vi "SUB-FILE-Measurement data_Load.vi"(7 "File Name":string="Temperature", 8 "File Server Path":string="C:\\InLCT\\Measurement Data\\WB1\\1111\\PT") -> (1 "배열-Data":dbl[][](array[numeric])=[[30.4, 28.4, 28.4, 28.4, 28.4, 28.4, 28.4, 28.4, 28.4, 28.4, 28.4, 28.4, 28.4, 28.4, 28.4, 28.4, 28.4, 28.4, 28.4, 28.4, 28.4, 28.4, 28.4, 28.4, 28.4, 28.4, 28.4, 28.4, 28.4, 28.4, 28.4, 28.4, 28.4, 28.4, 28.4, 28.4, 28.4, 28.4, 28.4, 28.4, 28.4, 28.4, 28.4, 28.4, 28.4, 28.4, 28.4, 28.4, 28.4, 28.4, 28.4, 28.4, 28.4, 28.4, 28.4, 28.4, 28.4, 28.4, 28.4, 28.4, 28.4, 28.4, 28.4, 28.4, 28.4, 28.4, 28.4, 28.4, 28.4, 28.4, 28.4, 28.4, 28.4, 28.4, 28.4, 28.4, 28.4, 28.4, 28.4, 28.4, 28.4, 28.4, 28.4, 28.4, 28.4, 28.4, 28.4, 28.4, 28.4, 28.4, 28.4, 28.4, 28.4, 28.4, 28.4, 28.4, 28.4, 28.4, 28.4, 28.4, 28.4, 28.4, 28.4, 28.4, 28.4, 28.4, 28.4, 28.4, 28.4, 28.4, 28.4, 28.4, 28.4, 28.4, 28.4, 28.4, 28.4, 28.4, 28.4, 28.4, 28.4, 28.4, 28.4, 28.4, 28.4, 28.4, 28.4, 28.4, 28.4, 28.4, 28.4, 28.4, 28.4, 28.4, 28.4, 28.4, 28.4, 28.4, 28.4, 28.4, 28.4, 28.4, 28.4, 28.4, 28.4, 28.4, 28.4, 28.4, 28.4, 28.4, 28.4, 28.4, 28.4, 28.4, 28.4, 28.4, 28.4, 28.4, 28.4, 28.4, 28.4, 28.4, 28.4, 28.4, 28.4, 28.4, 28.4, 28.4, 28.4, 28.4, 28.4, 28.4, 28.4, 28.4, 28.4, 28.4, 28.4, 28.4, 28.4, 28.4, 28.4, 28.4, 28.4, 28.4, 28.4, 28.4, 28.4, 28.4, 28.4, 28.4, 28.4, 28.4, 28.4, 28.4, 28.4, 28.4, 28.4, 28.4, 28.4, 28.4, 28.4, 28.4, 28.4, 28.4, 28.4, 28.4, 28.4, 28.4, 28.4, 28.4, 28.4, 28.4, 28.4, 28.4, 28.4, 28.4, 28.4, 28.4, 28.4, 28.4, 28.4, 28.4, 28.4, 28.4, 28.4, 28.4, 28.4, 28.4, 28.4, 28.4, 28.4, 28.4, 28.4, 28.4, 28.4, 28.4, 28.4, 28.4, 28.4, 28.4, 28.4, 28.4, 28.4, 28.4, 28.4, 28.4, 28.4, 28.4, 28.4, 28.4, 28.4, 28.4, 28.4, 28.4, 28.4, 28.4, 28.4, 28.4, 28.4, 28.4, 28.4, 28.4, 28.4, 28.4, 28.4, 28.4, 28.4, 28.4, 28.4, 28.4, 28.4, 28.4, 28.4, 28.4, 28.4, 28.4, 28.4, 28.4, 28.4, 28.4, 28.4, 28.4, 28.4, 28.4, 28.4, 28.4, 28.4, 28.4], [28.4, 28.4, 28.4, 28.4, 28.4, 28.4, 28.4, 28.4, 28.4, 28.4, 28.4, 28.4, 28.4, 28.4, 28.4, 28.4, 28.4, 28.4, 28.4, 28.4, 28.4, 28.4, 28.4, 28.4, 28.4, 28.4, 28.4, 28.4, 28.4, 28.4, 28.4, 28.4, 28.4, 28.4, 28.4, 28.4, 28.4, 28.4, 28.4, 28.4, 28.4, 28.4, 28.4, 28.4, 28.4, 28.4, 28.4, 28.4, 28.4, 28.4, 28.4, 28.4, 28.4, 28.4, 28.4, 28.4, 28.4, 28.4, 28.4, 28.4, 28.4, 28.4, 28.4, 28.4, 28.4, 28.4, 28.4, 28.4, 28.4, 28.4, 28.4, 28.4, 28.4, 28.4, 28.4, 28.4, 28.4, 28.4, 28.4, 28.4, 28.4, 28.4, 28.4, 28.4, 28.4, 28.4, 28.4, 28.4, 28.4, 28.4, 28.4, 28.4, 28.4, 28.4, 28.4, 28.4, 28.4, 28.4, 28.4, 28.4, 28.4, 28.4, 28.4, 28.4, 28.4, 28.4, 28.4, 28.4, 28.4, 28.4, 28.4, 28.4, 28.4, 28.4, 28.4, 28.4, 28.4, 28.4, 28.4, 28.4, 28.4, 28.4, 28.4, 28.4, 28.4, 28.4, 28.4, 28.4, 28.4, 28.4, 28.4, 28.4, 28.4, 28.4, 28.4, 28.4, 28.4, 28.4, 28.4, 28.4, 28.4, 28.4, 28.4, 28.4, 28.4, 28.4, 28.4, 28.4, 28.4, 28.4, 28.4, 28.4, 28.4, 28.4, 28.4, 28.4, 28.4, 28.4, 28.4, 28.4, 28.4, 28.4, 28.4, 28.4, 28.4, 28.4, 28.4, 28.4, 28.4, 28.4, 28.4, 28.4, 28.4, 28.4, 28.4, 28.4, 28.4, 28.4, 28.4, 28.4, 28.4, 28.4, 28.4, 28.4, 28.4, 28.4, 28.4, 28.4, 28.4, 28.4, 28.4, 28.4, 28.4, 28.4, 28.4, 28.4, 28.4, 28.4, 28.4, 28.4, 28.4, 28.4, 28.4, 28.4, 28.4, 28.4, 28.4, 28.4, 28.4, 28.4, 28.4, 28.4, 28.4, 28.4, 28.4, 28.4, 28.4, 28.4, 28.4, 28.4, 28.4, 28.4, 28.4, 28.4, 28.4, 28.4, 28.4, 28.4, 28.4, 28.4, 28.4, 28.4, 28.4, 28.4, 28.4, 28.4, 28.4, 28.4, 28.4, 28.4, 28.4, 28.4, 28.4, 28.4, 28.4, 28.4, 28.4, 28.4, 28.4, 28.4, 28.4, 28.4, 28.4, 28.4, 28.4, 28.4, 28.4, 28.4, 28.4, 28.4, 28.4, 28.4, 28.4, 28.4, 28.4, 28.4, 28.4, 28.4, 28.4, 28.4, 28.4, 28.4, 28.4, 28.4, 28.4, 28.4, 28.4, 28.4, 28.4, 28.4, 28.4, 28.4, 28.4, 28.4, 28.4, 28.4, 28.4, 28.4], [28.4, 28.4, 28.4, 28.4, 28.4, 28.4, 28.4, 28.4, 28.4, 28.4, 28.4, 28.4, 28.4, 28.4, 28.4, 28.4, 28.4, 28.4, 28.4, 28.4, 28.4, 28.4, 28.4, 28.4, 28.4, 28.4, 28.4, 28.4, 28.4, 28.4, 28.4, 28.4, 28.4, 28.4, 28.4, 28.4, 28.4, 28.4, 28.4, 28.4, 28.4, 28.4, 28.4, 28.4, 28.4, 28.4, 28.4, 28.4, 28.4, 28.4, 28.4, 28.4, 28.4, 28.4, 28.4, 28.4, 28.4, 28.4, 28.4, 28.4, 28.4, 28.4, 28.4, 28.4, 28.4, 28.4, 28.4, 28.4, 28.4, 28.4, 28.4, 28.4, 28.4, 28.4, 28.4, 28.4, 28.4, 28.4, 28.4, 28.4, 28.4, 28.4, 28.4, 28.4, 28.4, 28.4, 28.4, 28.4, 28.4, 28.4, 28.4, 28.4, 28.4, 28.4, 28.4, 28.4, 28.4, 28.4, 28.4, 28.4, 28.4, 28.4, 28.4, 28.4, 28.4, 28.4, 28.4, 28.4, 28.4, 28.4, 28.4, 28.4, 28.4, 28.4, 28.4, 28.4, 28.4, 28.4, 28.4, 28.4, 28.4, 28.4, 28.4, 28.4, 28.4, 28.4, 28.4, 28.4, 28.4, 28.4, 28.4, 28.4, 28.4, 28.4, 28.4, 28.4, 28.4, 28.4, 28.4, 28.4, 28.4, 28.4, 28.4, 28.4, 28.4, 28.4, 28.4, 28.4, 28.4, 28.4, 28.4, 28.4, 28.4, 28.4, 28.4, 28.4, 28.4, 28.4, 28.4, 28.4, 28.4, 28.4, 28.4, 28.4, 28.4, 28.4, 28.4, 28.4, 28.4, 28.4, 28.4, 28.4, 28.4, 28.4, 28.4, 28.4, 28.4, 28.4, 28.4, 28.4, 28.4, 28.4, 28.4, 28.4, 28.4, 28.4, 28.4, 28.4, 28.4, 28.4, 28.4, 28.4, 28.4, 28.4, 28.4, 28.4, 28.4, 28.4, 28.4, 28.4, 28.4, 28.4, 28.4, 28.4, 28.4, 28.4, 28.4, 28.4, 28.4, 28.4, 28.4, 28.4, 28.4, 28.4, 28.4, 28.4, 28.4, 28.4, 28.4, 28.4, 28.4, 28.4, 28.4, 28.4, 28.4, 28.4, 28.4, 28.4, 28.4, 28.4, 28.4, 28.4, 28.4, 28.4, 28.4, 28.4, 28.4, 28.4, 28.4, 28.4, 28.4, 28.4, 28.4, 28.4, 28.4, 28.4, 28.4, 28.4, 28.4, 28.4, 28.4, 28.4, 28.4, 28.4, 28.4, 28.4, 28.4, 28.4, 28.4, 28.4, 28.4, 28.4, 28.4, 28.4, 28.4, 28.4, 28.4, 28.4, 28.4, 28.4, 28.4, 28.4, 28.4, 28.4, 28.4, 28.4, 28.4, 28.4, 28.4, 28.4, 28.4, 28.4, 28.4, 28.4, 28.4, 28.4, 28.4, 28.4], [28.4, 28.4, 28.4, 28.4, 28.4, 28.4, 28.4, 28.4, 28.4, 28.4, 28.4, 28.4, 28.4, 28.4, 28.4, 28.4, 28.4, 28.4, 28.4, 28.4, 28.4, 28.4, 28.4, 28.4, 28.4, 28.4, 28.4, 28.4, 28.4, 28.4, 28.4, 28.4, 28.4, 28.4, 28.4, 28.4, 28.4, 28.4, 28.4, 28.4, 28.4, 28.4, 28.4, 28.4, 28.4, 28.4, 28.4, 28.4, 28.4, 28.4, 28.4, 28.4, 28.4, 28.4, 28.4, 28.4, 28.4, 28.4, 28.4, 28.4, 28.4, 28.4, 28.4, 28.4, 28.4, 28.4, 28.4, 28.4, 28.4, 28.4, 28.4, 28.4, 28.4, 28.4, 28.4, 28.4, 28.4, 28.4, 28.4, 28.4, 28.4, 28.4, 28.4, 28.4, 28.4, 28.4, 28.4, 28.4, 28.4, 28.4, 28.4, 28.4, 28.4, 28.4, 28.4, 28.4, 28.4, 28.4, 28.4, 28.4, 28.4, 28.4, 28.4, 28.4, 28.4, 28.4, 28.4, 28.4, 28.4, 28.4, 28.4, 28.4, 28.4, 28.4, 28.4, 28.4, 28.4, 28.4, 28.4, 28.4, 28.4, 28.4, 28.4, 28.4, 28.4, 28.4, 28.4, 28.4, 28.4, 28.4, 28.4, 28.4, 28.4, 28.4, 28.4, 28.4, 28.4, 28.4, 28.4, 28.4, 28.4, 28.4, 28.4, 28.4, 28.4, 28.4, 28.4, 28.4, 28.4, 28.4, 28.4, 28.4, 28.4, 28.4, 28.4, 28.4, 28.4, 28.4, 28.4, 28.4, 28.4, 28.4, 28.4, 28.4, 28.4, 28.4, 28.4, 28.4, 28.4, 28.4, 28.4, 28.4, 28.4, 28.4, 28.4, 28.4, 28.4, 28.4, 28.4, 28.4, 28.4, 28.4, 28.4, 28.4, 28.4, 28.4, 28.4, 28.4, 28.4, 28.4, 28.4, 28.4, 28.4, 28.4, 28.4, 28.4, 28.4, 28.4, 28.4, 28.4, 28.4, 28.4, 28.4, 28.4, 28.4, 28.4, 28.4, 28.4, 28.4, 28.4, 28.4, 28.4, 28.4, 28.4, 28.4, 28.4, 28.4, 28.4, 28.4, 28.4, 28.4, 28.4, 28.4, 28.4, 28.4, 28.4, 28.4, 28.4, 28.4, 28.4, 28.4, 28.4, 28.4, 28.4, 28.4, 28.4, 28.4, 28.4, 28.4, 28.4, 28.4, 28.4, 28.4, 28.4, 28.4, 28.4, 28.4, 28.4, 28.4, 28.4, 28.4, 28.4, 28.4, 28.4, 28.4, 28.4, 28.4, 28.4, 28.4, 28.4, 28.4, 28.4, 28.4, 28.4, 28.4, 28.4, 28.4, 28.4, 28.4, 28.4, 28.4, 28.4, 28.4, 28.4, 28.4, 28.4, 28.4, 28.4, 28.4, 28.4, 28.4, 28.4, 28.4, 28.4, 28.4, 28.4, 28.4, 28.4], [28.4, 28.4, 28.4, 28.4, 28.4, 28.4, 28.4, 28.4, 28.4, 28.4, 28.4, 28.4, 28.4, 28.4, 28.4, 28.4, 28.4, 28.4, 28.4, 28.4, 28.4, 28.4, 28.4, 28.4, 28.4, 28.4, 28.4, 28.4, 28.4, 28.4, 28.4, 28.4, 28.4, 28.4, 28.4, 28.4, 28.4, 28.4, 28.4, 28.4, 28.4, 28.4, 28.4, 28.4, 28.4, 28.4, 28.4, 28.4, 28.4, 28.4, 28.4, 28.4, 28.4, 28.4, 28.4, 28.4, 28.4, 28.4, 28.4, 28.4, 28.4, 28.4, 28.4, 28.4, 28.4, 28.4, 28.4, 28.4, 28.4, 28.4, 28.4, 28.4, 28.4, 28.4, 28.4, 28.4, 28.4, 28.4, 28.4, 28.4, 28.4, 28.4, 28.4, 28.4, 28.4, 28.4, 28.4, 28.4, 28.4, 28.4, 28.4, 28.4, 28.4, 28.4, 28.4, 28.4, 28.4, 28.4, 28.4, 28.4, 28.4, 28.4, 28.4, 28.4, 28.4, 28.4, 28.4, 28.4, 28.4, 28.4, 28.4, 28.4, 28.4, 28.4, 28.4, 28.4, 28.4, 28.4, 28.4, 28.4, 28.4, 28.4, 28.4, 28.4, 28.4, 28.4, 28.4, 28.4, 28.4, 28.4, 28.4, 28.4, 28.4, 28.4, 28.4, 28.4, 28.4, 28.4, 28.4, 28.4, 28.4, 28.4, 28.4, 28.4, 28.4, 28.4, 28.4, 28.4, 28.4, 28.4, 28.4, 28.4, 28.4, 28.4, 28.4, 28.4, 28.4, 28.4, 28.4, 28.4, 28.4, 28.4, 28.4, 28.4, 28.4, 28.4, 28.4, 28.4, 28.4, 28.4, 28.4, 28.4, 28.4, 28.4, 28.4, 28.4, 28.4, 28.4, 28.4, 28.4, 28.4, 28.4, 28.4, 28.4, 28.4, 28.4, 28.4, 28.4, 28.4, 28.4, 28.4, 28.4, 28.4, 28.4, 28.4, 28.4, 28.4, 28.4, 28.4, 28.4, 28.4, 28.4, 28.4, 28.4, 28.4, 28.4, 28.4, 28.4, 28.4, 28.4, 28.4, 28.4, 28.4, 28.4, 28.4, 28.4, 28.4, 28.4, 28.4, 28.4, 28.4, 28.4, 28.4, 28.4, 28.4, 28.4, 28.4, 28.4, 28.4, 28.4, 28.4, 28.4, 28.4, 28.4, 28.4, 28.4, 28.4, 28.4, 28.4, 28.4, 28.4, 28.4, 28.4, 28.4, 28.4, 28.4, 28.4, 28.4, 28.4, 28.4, 28.4, 28.4, 28.4, 28.4, 28.4, 28.4, 28.4, 28.4, 28.4, 28.4, 28.4, 28.4, 28.4, 28.4, 28.4, 28.4, 28.4, 28.4, 28.4, 28.4, 28.4, 28.4, 28.4, 28.4, 28.4, 28.4, 28.4, 28.4, 28.4, 28.4, 28.4, 28.4, 28.4, 28.4, 28.4, 28.4, 28.4, 28.4], [28.4, 28.4, 28.4, 28.4, 28.4, 28.4, 28.4, 28.4, 28.4, 28.4, 28.4, 28.4, 28.4, 28.4, 28.4, 28.4, 28.4, 28.4, 28.4, 28.4, 28.4, 28.4, 28.4, 28.4, 28.4, 28.4, 28.4, 28.4, 28.4, 28.4, 28.4, 28.4, 28.4, 28.4, 28.4, 28.4, 28.4, 28.4, 28.4, 28.4, 28.4, 28.4, 28.4, 28.4, 28.4, 28.4, 28.4, 28.4, 28.4, 28.4, 28.4, 28.4, 28.4, 28.4, 28.4, 28.4, 28.4, 28.4, 28.4, 28.4, 28.4, 28.4, 28.4, 28.4, 28.4, 28.4, 28.4, 28.4, 28.4, 28.4, 28.4, 28.4, 28.4, 28.4, 28.4, 28.4, 28.4, 28.4, 28.4, 28.4, 28.4, 28.4, 28.4, 28.4, 28.4, 28.4, 28.4, 28.4, 28.4, 28.4, 28.4, 28.4, 28.4, 28.4, 28.4, 28.4, 28.4, 28.4, 28.4, 28.4, 28.4, 28.4, 28.4, 28.4, 28.4, 28.4, 28.4, 28.4, 28.4, 28.4, 28.4, 28.4, 28.4, 28.4, 28.4, 28.4, 28.4, 28.4, 28.4, 28.4, 28.4, 28.4, 28.4, 28.4, 28.4, 28.4, 28.4, 28.4, 28.4, 28.4, 28.4, 28.4, 28.4, 28.4, 28.4, 28.4, 28.4, 28.4, 28.4, 28.4, 28.4, 28.4, 28.4, 28.4, 28.4, 28.4, 28.4, 28.4, 28.4, 28.4, 28.4, 28.4, 28.4, 28.4, 28.4, 28.4, 28.4, 28.4, 28.4, 28.4, 28.4, 28.4, 28.4, 28.4, 28.4, 28.4, 28.4, 28.4, 28.4, 28.4, 28.4, 28.4, 28.4, 28.4, 28.4, 28.4, 28.4, 28.4, 28.4, 28.4, 28.4, 28.4, 28.4, 28.4, 28.4, 28.4, 28.4, 28.4, 28.4, 28.4, 28.4, 28.4, 28.4, 28.4, 28.4, 28.4, 28.4, 28.4, 28.4, 28.4, 28.4, 28.4, 28.4, 28.4, 28.4, 28.4, 28.4, 28.4, 28.4, 28.4, 28.4, 28.4, 28.4, 28.4, 28.4, 28.4, 28.4, 28.4, 28.4, 28.4, 28.4, 28.4, 28.4, 28.4, 28.4, 28.4, 28.4, 28.4, 28.4, 28.4, 28.4, 28.4, 28.4, 28.4, 28.4, 28.4, 28.4, 28.4, 28.4, 28.4, 28.4, 28.4, 28.4, 28.4, 28.4, 28.4, 28.4, 28.4, 28.4, 28.4, 28.4, 28.4, 28.4, 28.4, 28.4, 28.4, 28.4, 28.4, 28.4, 28.4, 28.4, 28.4, 28.4, 28.4, 28.4, 28.4, 28.4, 28.4, 28.4, 28.4, 28.4, 28.4, 28.4, 28.4, 28.4, 28.4, 28.4, 28.4, 28.4, 28.4, 28.4, 28.4, 28.4, 28.4, 28.4, 28.4, 28.4, 28.4], [28.4, 28.4, 28.4, 28.4, 28.4, 28.4, 28.4, 28.4, 28.4, 28.4, 28.4, 28.4, 28.4, 28.4, 28.4, 28.4, 28.4, 28.4, 28.4, 28.4, 28.4, 28.4, 28.4, 28.4, 28.4, 28.4, 28.4, 28.4, 28.4, 28.4, 28.4, 28.4, 28.4, 28.4, 28.4, 28.4, 28.4, 28.4, 28.4, 28.4, 28.4, 28.4, 28.4, 28.4, 28.4, 28.4, 28.4, 28.4, 28.4, 28.4, 28.4, 28.4, 28.4, 28.4, 28.4, 28.4, 28.4, 28.4, 28.4, 28.4, 28.4, 28.4, 28.4, 28.4, 28.4, 28.4, 28.4, 28.4, 28.4, 28.4, 28.4, 28.4, 28.4, 28.4, 28.4, 28.4, 28.4, 28.4, 28.4, 28.4, 28.4, 28.4, 28.4, 28.4, 28.4, 28.4, 28.4, 28.4, 28.4, 28.4, 28.4, 28.4, 28.4, 28.4, 28.4, 28.4, 28.4, 28.4, 28.4, 28.4, 28.4, 28.4, 28.4, 28.4, 28.4, 28.4, 28.4, 28.4, 28.4, 28.4, 28.4, 28.4, 28.4, 28.4, 28.4, 28.4, 28.4, 28.4, 28.4, 28.4, 28.4, 28.4, 28.4, 28.4, 28.4, 28.4, 28.4, 28.4, 28.4, 28.4, 28.4, 28.4, 28.4, 28.4, 28.4, 28.4, 28.4, 28.4, 28.4, 28.4, 28.4, 28.4, 28.4, 28.4, 28.4, 28.4, 28.4, 28.4, 28.4, 28.4, 28.4, 28.4, 28.4, 28.4, 28.4, 28.4, 28.4, 28.4, 28.4, 28.4, 28.4, 28.4, 28.4, 28.4, 28.4, 28.4, 28.4, 28.4, 28.4, 28.4, 28.4, 28.4, 28.4, 28.4, 28.4, 28.4, 28.4, 28.4, 28.4, 28.4, 28.4, 28.4, 28.4, 28.4, 28.4, 28.4, 28.4, 28.4, 28.4, 28.4, 28.4, 28.4, 28.4, 28.4, 28.4, 28.4, 28.4, 28.4, 28.4, 28.4, 28.4, 28.4, 28.4, 28.4, 28.4, 28.4, 28.4, 28.4, 28.4, 28.4, 28.4, 28.4, 28.4, 28.4, 28.4, 28.4, 28.4, 28.4, 28.4, 28.4, 28.4, 28.4, 28.4, 28.4, 28.4, 28.4, 28.4, 28.4, 28.4, 28.4, 28.4, 28.4, 28.4, 28.4, 28.4, 28.4, 28.4, 28.4, 28.4, 28.4, 28.4, 28.4, 28.4, 28.4, 28.4, 28.4, 28.4, 28.4, 28.4, 28.4, 28.4, 28.4, 28.4, 28.4, 28.4, 28.4, 28.4, 28.4, 28.4, 28.4, 28.4, 28.4, 28.4, 28.4, 28.4, 28.4, 28.4, 28.4, 28.4, 28.4, 28.4, 28.4, 28.4, 28.4, 28.4, 28.4, 28.4, 28.4, 28.4, 28.4, 28.4, 28.4, 28.4, 28.4, 28.4, 28.4, 28.4, 28.4], [28.4, 28.4, 28.4, 28.4, 28.4, 28.4, 28.4, 28.4, 28.4, 28.4, 28.4, 28.4, 28.4, 28.4, 28.4, 28.4, 28.4, 28.4, 28.4, 28.4, 28.4, 28.4, 28.4, 28.4, 28.4, 28.4, 28.4, 28.4, 28.4, 28.4, 28.4, 28.4, 28.4, 28.4, 28.4, 28.4, 28.4, 28.4, 28.4, 28.4, 28.4, 28.4, 28.4, 28.4, 28.4, 28.4, 28.4, 28.4, 28.4, 28.4, 28.4, 28.4, 28.4, 28.4, 28.4, 28.4, 28.4, 28.4, 28.4, 28.4, 28.4, 28.4, 28.4, 28.4, 28.4, 28.4, 28.4, 28.4, 28.4, 28.4, 28.4, 28.4, 28.4, 28.4, 28.4, 28.4, 28.4, 28.4, 28.4, 28.4, 28.4, 28.4, 28.4, 28.4, 28.4, 28.4, 28.4, 28.4, 28.4, 28.4, 28.4, 28.4, 28.4, 28.4, 28.4, 28.4, 28.4, 28.4, 28.4, 28.4, 28.4, 28.4, 28.4, 28.4, 28.4, 28.4, 28.4, 28.4, 28.4, 28.4, 28.4, 28.4, 28.4, 28.4, 28.4, 28.4, 28.4, 28.4, 28.4, 28.4, 28.4, 28.4, 28.4, 28.4, 28.4, 28.4, 28.4, 28.4, 28.4, 28.4, 28.4, 28.4, 28.4, 28.4, 28.4, 28.4, 28.4, 28.4, 28.4, 28.4, 28.4, 28.4, 28.4, 28.4, 28.4, 28.4, 28.4, 28.4, 28.4, 28.4, 28.4, 28.4, 28.4, 28.4, 28.4, 28.4, 28.4, 28.4, 28.4, 28.4, 28.4, 28.4, 28.4, 28.4, 28.4, 28.4, 28.4, 28.4, 28.4, 28.4, 28.4, 28.4, 28.4, 28.4, 28.4, 28.4, 28.4, 28.4, 28.4, 28.4, 28.4, 28.4, 28.4, 28.4, 28.4, 28.4, 28.4, 28.4, 28.4, 28.4, 28.4, 28.4, 28.4, 28.4, 28.4, 28.4, 28.4, 28.4, 28.4, 28.4, 28.4, 28.4, 28.4, 28.4, 28.4, 28.4, 28.4, 28.4, 28.4, 28.4, 28.4, 28.4, 28.4, 28.4, 28.4, 28.4, 28.4, 28.4, 28.4, 28.4, 28.4, 28.4, 28.4, 28.4, 28.4, 28.4, 28.4, 28.4, 28.4, 28.4, 28.4, 28.4, 28.4, 28.4, 28.4, 28.4, 28.4, 28.4, 28.4, 28.4, 28.4, 28.4, 28.4, 28.4, 28.4, 28.4, 28.4, 28.4, 28.4, 28.4, 28.4, 28.4, 28.4, 28.4, 28.4, 28.4, 28.4, 28.4, 28.4, 28.4, 28.4, 28.4, 28.4, 28.4, 28.4, 28.4, 28.4, 28.4, 28.4, 28.4, 28.4, 28.4, 28.4, 28.4, 28.4, 28.4, 28.4, 28.4, 28.4, 28.4, 28.4, 28.4, 28.4, 28.4, 28.4, 28.4, 28.4, 28.4]], 2 "배열-열헤더":string[](array[string])=["1", "1", "1", "1", "1", "1", "1", "1"], 3 "정상(T)":bool caption="정상")   [LabVIEW 2015]
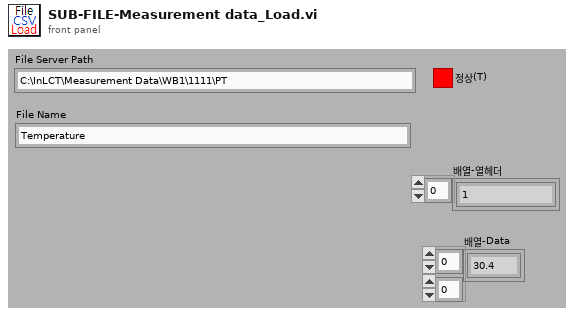
[diagram p1: front panel]
types:
  T1 = enum16{"open", "replace", "create", "open or create", "replace or create", "replace or create with confirmation"}
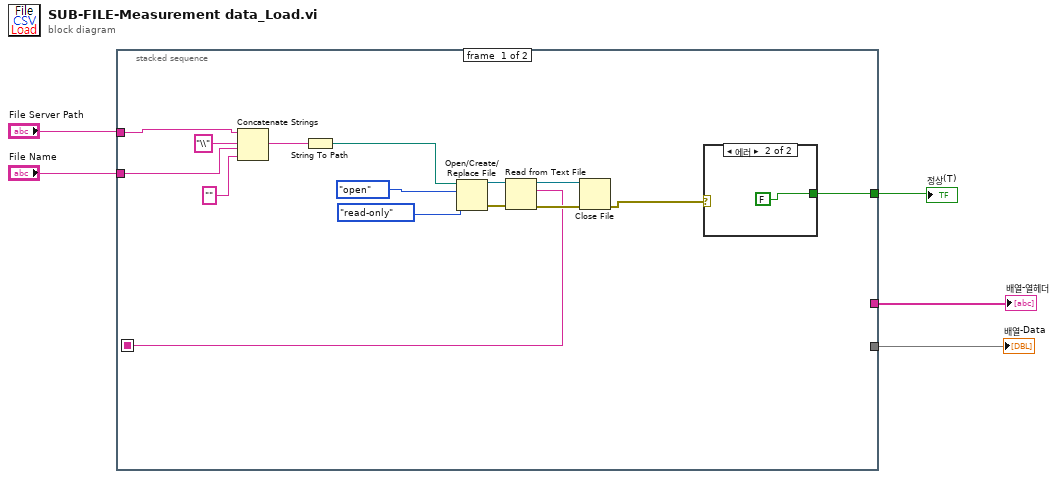
[diagram p0: block diagram]
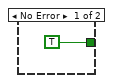
[diagram p2: hidden frame]
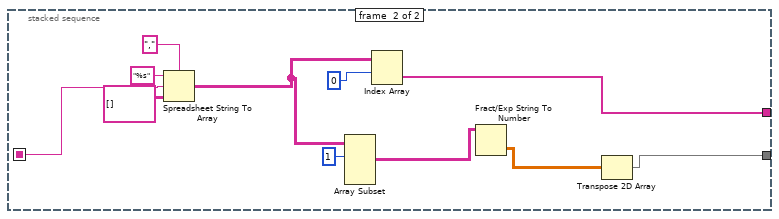
[diagram p3: hidden frame]
diagram:
  n1 = stacked-sequence {
    seq-local: [w6 _] -> [_ w32]
    tunnel: "File Server Path" -> [w18 _]
    tunnel: "File Name" -> [w17 _]
    tunnel: [w16 _] -> w3
    tunnel: [_ w29] -> w2
    tunnel: [_ w23] -> w1
    frame #0 {
      n2 = Concatenate Strings(w18, "\\" ("format (%.3f)"), w17, "" ("format (%.3f)")) -> (w19:string)
      n3 = String To Path(string=w19) -> (path=w7:path)
      n4 = Open/Create/Replace File(file path (use dialog)=w7, operation (0:open)=T1."open" ("동작(0:open)"), access (0:read/write)=enum16{"read/write", "read-only", "write-only"}."read-only" ("접근(0:읽기/쓰기)")) -> (refnum out=w11:refnum<file>, error out=w12:errorcluster)  [unwired: 1 in, 3 out]
      n5 = Read from Text File(file (use dialog)=w11, error in=w12) -> (refnum out=w14:refnum<file>, text=w6:string, error out=w13:errorcluster)  [unwired: 3 out]
      n6 = Close File(refnum=w14, error in=w13) -> (error out=w8:errorcluster)  [unwired: 1 out]
      n7 = case shown="에러" w8 {
        tunnel: [TRUE FALSE] -> w16
        frame No Error {
        }
        frame Error {
        }
      }
    }
    frame #1 {
      n8 = Spreadsheet String To Array(delimiter (Tab)="," ("구분 문자(탭)"), format string="%s" ("포맷 문자열"), spreadsheet string=w32, array type (2D Dbl)=string[][] [] ("배열 타입(2D Dbl)")) -> (array=w27:string[][])
      n9 = Array Subset(array=w27, index (row)=1 ("인덱스")) -> (w25:string[][])  [unwired: 3 in]
      n10 = Index Array(array=w27, index (row)=0 ("비활성화된 인덱스 (열)")) -> (element=w29:string[])  [unwired: 1 in]
      n11 = Fract/Exp String To Number(string=w25) -> (number=w24:dbl[][])  [unwired: 3 in, 1 out]
      n12 = Transpose 2D Array(2D array=w24) -> (transposed array=w23:dbl[][])
    }
  }
  "배열-열헤더" <- w2
  "배열-Data" <- w1
  "정상(T)" <- w3
